vi "Init_DAQ_tasks_NI.vi"(6 "error in":errorcluster, 9 "Device parameters":T1 {"Read chunk size" min=100 max=100000; "Acquisition sample rate" min=10.0 max=10000.0 step=10.0; "Stimulation sample rate" min=10.0 max=10000.0}) -> (0 "error out":errorcluster, 3 "DAQ task out":refnum<k21>)   [LabVIEW 2010]
uses:
  typedefs/device_parameters.ctl
  <vilib>/DAQmx/create/channels.llb/DAQmx Create Channel (AI-Voltage-Basic).vi
  <vilib>/DAQmx/configure/timing.llb/DAQmx Timing (Sample Clock).vi
  <vilib>/DAQmx/configure/trigger.llb/DAQmx Start Trigger (Digital Edge).vi
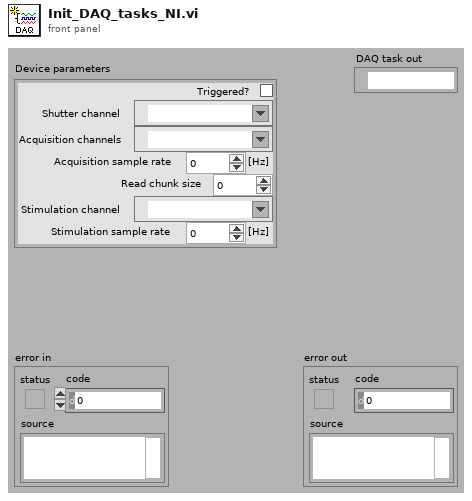
[diagram p1: front panel]
types:
  T1 = typedef "device_parameters.ctl" = cluster{"Triggered?":bool, "Shutter channel":tag, "Acquisition channels":tag, "Acquisition sample rate":dbl, "Read chunk size":i32, "Stimulation channel":tag, "Stimulation sample rate":dbl}
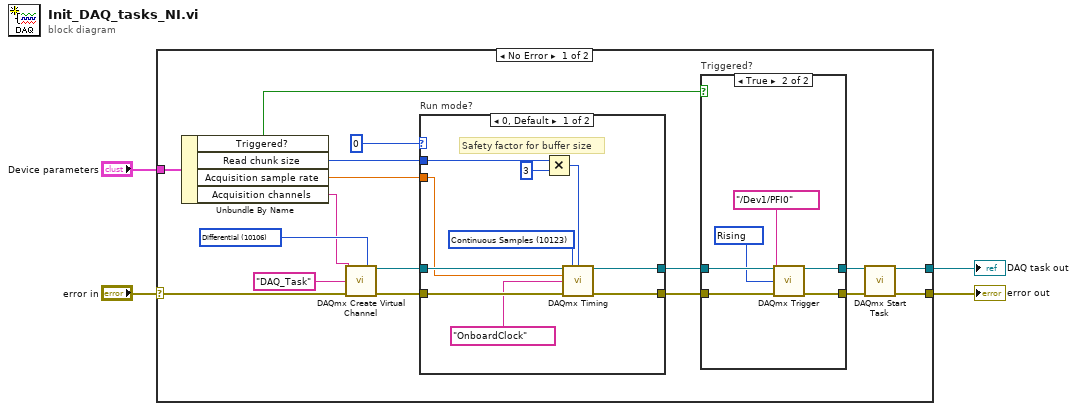
[diagram p0: block diagram]
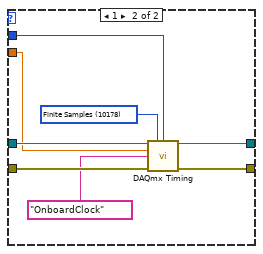
[diagram p2: hidden frame]
diagram:
  n1 = case shown="No Error" "error in" {
    selector: "error in" -> [w12 w48]
    tunnel: [w8 w48] -> w4
    tunnel: "Device parameters" -> [w13 _]
    tunnel: [w6 _] -> w2
    frame No Error {
      w10 = 10106 items=["default"=-1, "RSE"=10083, "NRSE"=10078, "Differential"=10106, "Pseudodifferential"=12529] ("input terminal configuration")
      n2 = Unbundle By Name(w13) -> ("Triggered?"=w18:bool, "Read chunk size"=w17:i32, "Acquisition sample rate"=w19:dbl, "Acquisition channels"=w5:tag)
      n3 = call-poly <vilib>:"DAQmx Create Virtual Channel.vi"("input terminal configuration"=w10, "physical channels"=w5, "name to assign"="DAQ_Task", "error in"=w12) -> ("task out"=w14:refnum<k21>, "error out"=w16:errorcluster)  [unwired: 10 in]
      n4 = case "Run mode?" shown="0, Default" 0 ("Write chunk size") {
        tunnel: [w24 w37] -> w21
        tunnel: [w30 w38] -> w20
        tunnel: w19 -> [w22 w33]
        tunnel: w16 -> [w31 w39]
        tunnel: w17 -> [w26 w32]
        tunnel: w14 -> [w29 w36]
        frame 0, Default {
          w27 = 10123 items=["Finite Samples"=10178, "Continuous Samples"=10123, "Hardware Timed Single Point"=12522] ("sample mode")
          # "Safety factor for buffer size"
          n5 = Multiply(x=w26, y=3) -> (x*y=w23:i32)
          n6 = call-poly <vilib>:"DAQmx Timing.vi"("task/channels in"=w29, "sample mode"=w27, "samples per channel"=w23, "rate"=w22, "source"=tag "OnboardClock", "error in"=w31) -> ("task out"=w24:refnum<k21>, "error out"=w30:errorcluster)  [unwired: 8 in]
        }
        frame 1 {
          w34 = 10178 items=["Finite Samples"=10178, "Continuous Samples"=10123, "Hardware Timed Single Point"=12522] ("sample mode")
          n7 = call-poly <vilib>:"DAQmx Timing.vi"("task/channels in"=w36, "sample mode"=w34, "samples per channel"=w32, "rate"=w33, "source"=tag "OnboardClock", "error in"=w39) -> ("task out"=w37:refnum<k21>, "error out"=w38:errorcluster)  [unwired: 8 in]
        }
      }
      n8 = case "Triggered?" shown="True" w18 {
        tunnel: w20 -> [w40 w47]
        tunnel: [w40 w46] -> w9
        tunnel: w21 -> [w41 w45]
        tunnel: [w41 w44] -> w7
        frame False {
        }
        frame True {
          w42 = 10280 items=["Rising"=10280, "Falling"=10171] ("edge")
          n9 = call-poly <vilib>:"DAQmx Trigger.vi"("task/channels in"=w45, "source"=tag "/Dev1/PFI0", "edge"=w42, "error in"=w47) -> ("task out"=w44:refnum<k21>, "error out"=w46:errorcluster)  [unwired: 10 in]
        }
      }
      n10 = call <vilib>:"DAQmx Start Task.vi"("task/channels in"=w7, "error in"=w9) -> ("task out"=w6:refnum<k21>, "error out"=w8:errorcluster)  [unwired: 12 in]
    }
    frame Error {
    }
  }
  "error out" <- w4
  "DAQ task out" <- w2
